vi "Configure Detector Bandwidth.vi"(7 "Bandwidth (1: 30Hz)":i32(ring)=1 items=["3Hz", "30Hz", "300Hz"], 8 "error in (no error)":errorcluster, 9 "Channel List(\"\")":string, 10 "Function (1: Voltage AC)":i32(ring)=1 items=["Voltage AC"=1, "Current AC"=3], 11 "VISA resource name":refnum<visa-resource-name>) -> (0 "error out":errorcluster, 3 "VISA resource name out":refnum<visa-resource-name>)   [LabVIEW 2023, in "Keithley DMM6500 DAQ6500 Series.lvlib"]
doc: "Selects the detector bandwidth for AC current and AC voltage measurements."
uses:
  <instrlib>/Keithley DMM6500 DAQ6500 Series/Keithley DMM6500 DAQ6500 Series.lvlib
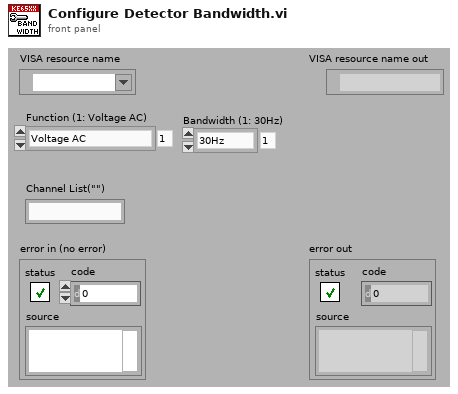
[diagram p1: front panel]
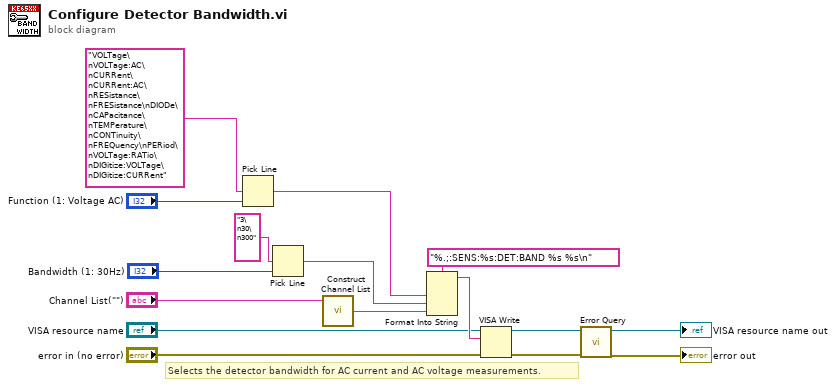
[diagram p0: block diagram]
diagram:
  # "Selects the detector bandwidth for AC current and AC voltage measurements."
  n1 = Pick Line(multi-line string="VOLTage\nVOLTage:AC\nCURRent\nCURRent:AC\nRESistance\nFRESistance\nDIODe\nCAPacitance\nTEMPerature\nCONTinuity\nFREQuency\nPERiod\nVOLTage:RATio\nDIGitize:VOLTage\nDIGitize:CURRent", line index="Function (1: Voltage AC)") -> (output string=w5:string)  [unwired: 1 in]
  n2 = Pick Line(multi-line string="3\n30\n300", line index="Bandwidth (1: 30Hz)") -> (output string=w4:string)  [unwired: 1 in]
  n3 = call <instrlib>:"Construct Channel List.vi"("Channel List"="Channel List(\"\")") -> ("Channel List String"=w7:string)  [unwired: 2 in]
  n4 = Format Into String(format string="%.;:SENS:%s:DET:BAND %s %s\n", w5, w4, w7) -> (resulting string=w15:string)  [unwired: 2 in, 1 out]
  n5 = VISA Write(VISA resource name="VISA resource name", write buffer=w15, error in (no error)="error in (no error)") -> (VISA resource name out=w12:refnum<visa-resource-name>, error out=w11:errorcluster)  [unwired: 1 out]
  n6 = call <instrlib>:"Error Query.vi"("error in (no error)"=w11, "VISA resource name"=w12) -> ("error out"=→"error out":errorcluster, "VISA resource name out"=→"VISA resource name out":refnum<visa-resource-name>)  [unwired: 6 in, 2 out]
